vi "Thermal_runaway.vi"() -> ()   [LabVIEW 2017]
panel:
  out "Av T":dbl(graph)
  in  "stop":bool
  out "Power":sgl(graph)
  out "I/V":cluster{"Voltage":sgl, "Current":sgl}(graph)
  in  "?":dbl=5000.0 format="%#_13g"
  in  "Vini":dbl format="%#_13g"
  out "Power":dbl format="%#_4g"
  in  "VISA resource name":refnum<visa-resource-name>="GPIB0::24::INSTR"
  in  "Source Mode  (0: Voltage)":u16(ring) items=["Voltage", "Current"]
  in  "Compliance  Level (0.1)":dbl=1.05
  out "Av T":dbl format="%#.2g"
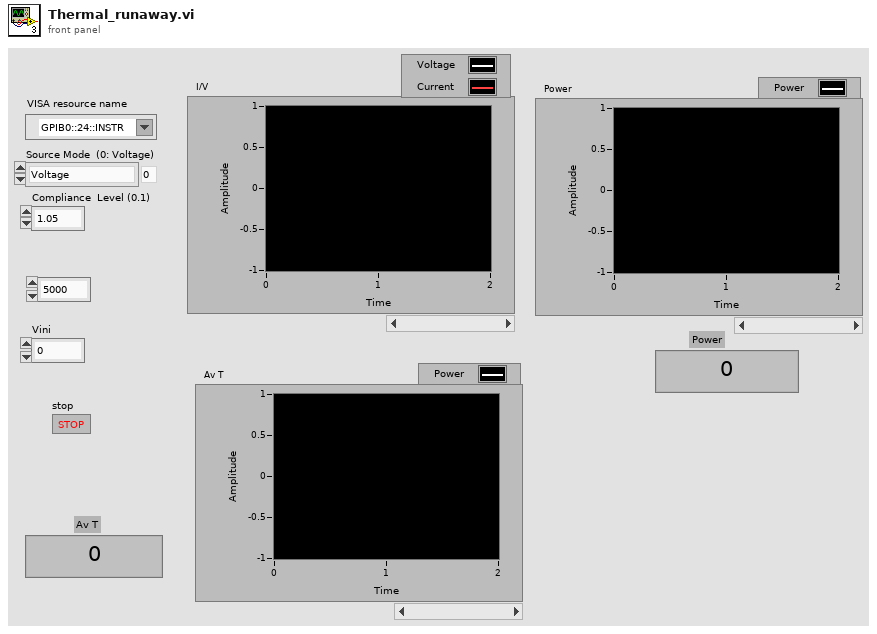
[diagram p1: front panel]
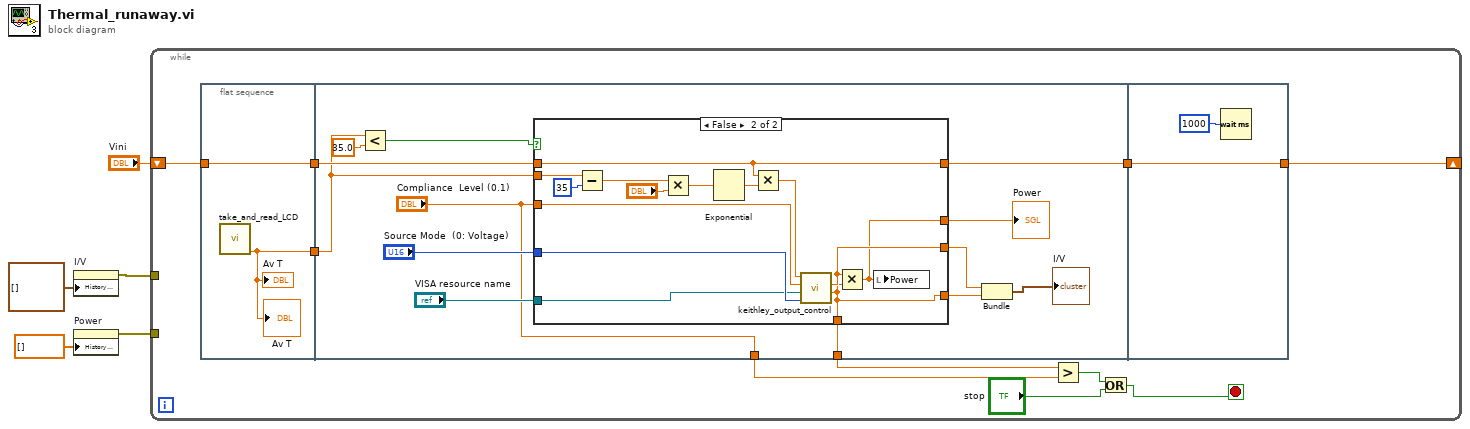
[diagram p0: block diagram]
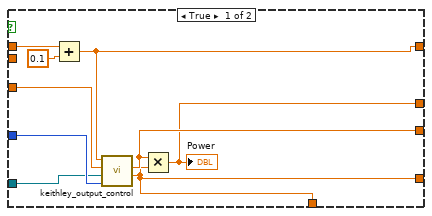
[diagram p2: hidden frame]
diagram:
  n1 = property on="I/V" class="WFChart (strict)"("History Data"=cluster{"Voltage":sgl, "Current":sgl}[] []) -> (error out=w3:errorcluster)  [unwired: 2 in, 1 out]
  n2 = property on="Power" class="WFChart (strict)"("History Data"=sgl[] []) -> (error out=w4:errorcluster)  [unwired: 2 in, 1 out]
  n3 = while {
    shift-right: [w12] -> _
    shift-left: "Vini" -> [w13]
    tunnel: w4 -> [_]
    tunnel: w3 -> [_]
    stop <- w7 stop-if-true
    n4 = flat-sequence {
      tunnel: [w16] -> w15
      tunnel: [w17] -> w14
      tunnel: w13 -> [w17]
      tunnel: w15 -> [w26]
      tunnel: w14 -> [w28]
      tunnel: [w27] -> w11
      tunnel: [w23] -> w10
      tunnel: ["Compliance  Level (0.1)"] -> w9
      tunnel: [w55] -> w12
      tunnel: w11 -> [w55]
      frame #0 {
        n5 = call "take_and_read_LCD.vi"() -> ("Av T"=w16:dbl)  [unwired: 9 in, 2 out]
        "Av T" <- w16
        "Av T" <- w16
      }
      frame #1 {
        n6 = Less?(x=w26, y=35.0) -> (x < y?=w29:bool)
        n7 = case shown="False" w29 {
          tunnel: w28 -> [w39 w46]
          tunnel: [w37 w46] -> w27
          tunnel: w26 -> [_ w48]
          tunnel: "Compliance  Level (0.1)" -> [w36 w43]
          tunnel: "Source Mode  (0: Voltage)" -> [w35 w45]
          tunnel: "VISA resource name" -> [w34 w44]
          tunnel: [w32 w41] -> w23
          tunnel: [w33 w42] -> w21
          tunnel: [w32 w41] -> w20
          tunnel: [w31 w40] -> w18
          frame True {
            n8 = Add(x=w39, y=0.1) -> (x+y=w37:dbl)
            n9 = call "keithley_output_control.vi"("Source Mode  (0: Voltage)"=w35, "VISA resource name"=w34, "Compliance  Level (0.1)"=w36, "Output Level (0)"=w37) -> ("Current"=w32:sgl, "Voltage"=w33:sgl)  [unwired: 5 in, 1 out]
            n10 = Multiply(x=w33, y=w32) -> (x*y=w31:sgl)
            "Power" <- w31
          }
          frame False {
            n11 = Subtract(x=w48, y=35) -> (x-y=w50:dbl)
            n12 = Multiply(x=w50, y="?") -> (x*y=w49:dbl)
            n13 = Exponential(1:w49) -> (0:w53:dbl)
            n14 = Multiply(x=w46, y=w53) -> (x*y=w52:dbl)
            n15 = call "keithley_output_control.vi"("Source Mode  (0: Voltage)"=w45, "VISA resource name"=w44, "Compliance  Level (0.1)"=w43, "Output Level (0)"=w52) -> ("Current"=w41:sgl, "Voltage"=w42:sgl)  [unwired: 5 in, 1 out]
            n16 = Multiply(x=w42, y=w41) -> (x*y=w40:sgl)
            n17 = local write "Power"(w40) -> ()
          }
        }
        "Power" <- w18
        n18 = Bundle("Voltage"=w21, "Current"=w20) -> (→"I/V":cluster{"Voltage":sgl, "Current":sgl})  [unwired: 1 in]
      }
      frame #2 {
        n19 = Wait (ms)(milliseconds to wait=u32 1000) -> ()  [unwired: 1 out]
      }
    }
    n20 = Greater?(x=w10, y=w9) -> (0:w8:bool)
    n21 = Or(x=w8, y="stop") -> (x .or. y?=w7:bool)
  }
